vi "PPMS.Get Magnet.vi"(8 "error in (no error)":errorcluster, 11 "instrument.PPMS":refnum<class "instrument.PPMS.lvclass">) -> (0 "error out":errorcluster, 2 "Magnet Status":T1, 3 "instrument.PPMS out":refnum<class "instrument.PPMS.lvclass">)   [LabVIEW 2019, in "instrument.PPMS.lvclass"]
uses:
  instrument.PPMS.lvclass
  Typedefs/PPMS.Magnet Status--cluster.ctl
  instrument.PPMS.lvclass/instrument.PPMS.ctl
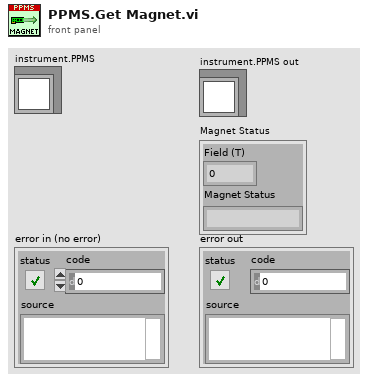
[diagram p1: front panel]
types:
  T1 = typedef "instrument.PPMS.lvclass/PPMS.Magnet Status--cluster.ctl" = cluster{"Field (T)":dbl, "Magnet Status":string}
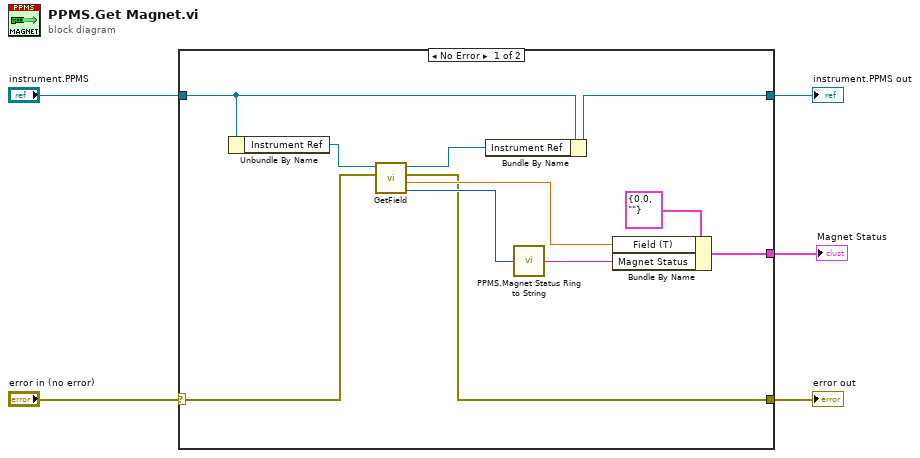
[diagram p0: block diagram]
diagram:
  n1 = case shown="No Error" "error in (no error)" {
    selector: "error in (no error)" -> [w6 w18]
    tunnel: [w8 w18] -> w5
    tunnel: "instrument.PPMS" -> [w11 w17]
    tunnel: [w12 w17] -> w2
    tunnel: [w15 _] -> w1
    frame No Error {
      n2 = Unbundle By Name(w11) -> ("Instrument Ref"=w14:refnum<k24>)
      n3 = call "GetField.vi"("error in (no error)"=w6, "Instrument Ref In"=w14) -> ("Field\nStatus"=w9:i32, "Field"=w10:dbl, "error out"=w8:errorcluster, "Instrument Ref Out"=w13:refnum<k24>)  [unwired: 3 in, 1 out]
      n4 = Bundle By Name(cluster=w11, "Instrument Ref"=w13) -> (w12:refnum<class "instrument.PPMS.lvclass">)
      n5 = call "PPMS.Magnet Status Ring to String.vi"("Field Status"=w9) -> ("Status String"=w7:string)
      n6 = Bundle By Name(cluster=T1 {"Field (T)"=0.0, "Magnet Status"=""} ("Magnet Status"), "Field (T)"=w10, "Magnet Status"=w7) -> (w15:T1)
    }
    frame Error {
    }
  }
  "Magnet Status" <- w1
  "error out" <- w5
  "instrument.PPMS out" <- w2
